vi "Check_Pos_R.vi"(0 "FPGA_Data":sgl[](array[numeric]), 2 "Q_MotorCmd_IN":refnum<queue>, 3 "Q_MotorCmd_Err_IN":errorcluster, 7 "Param_In":T1) -> (6 "LOAD_CELL_PEAK_R":sgl[](array[numeric]), 12 "Target_Pos":i32, 13 "Param_Out":T1, 14 "Flag":T2(ring), 15 "R_NUM":u32, 16 "Q_MotorCmd_OUT":refnum<queue>, 17 "Q_MotorCmd_Err_OUT":errorcluster, 18 "R_Period":u32, 19 "R_GCP":sgl)   [LabVIEW 2019]
uses:
  RT_GLOBAL.vi
panel:
  out "R_Period_EXT":u32
  out "R_GCP_EXT":sgl
  out "R_NUM_EXT":u32
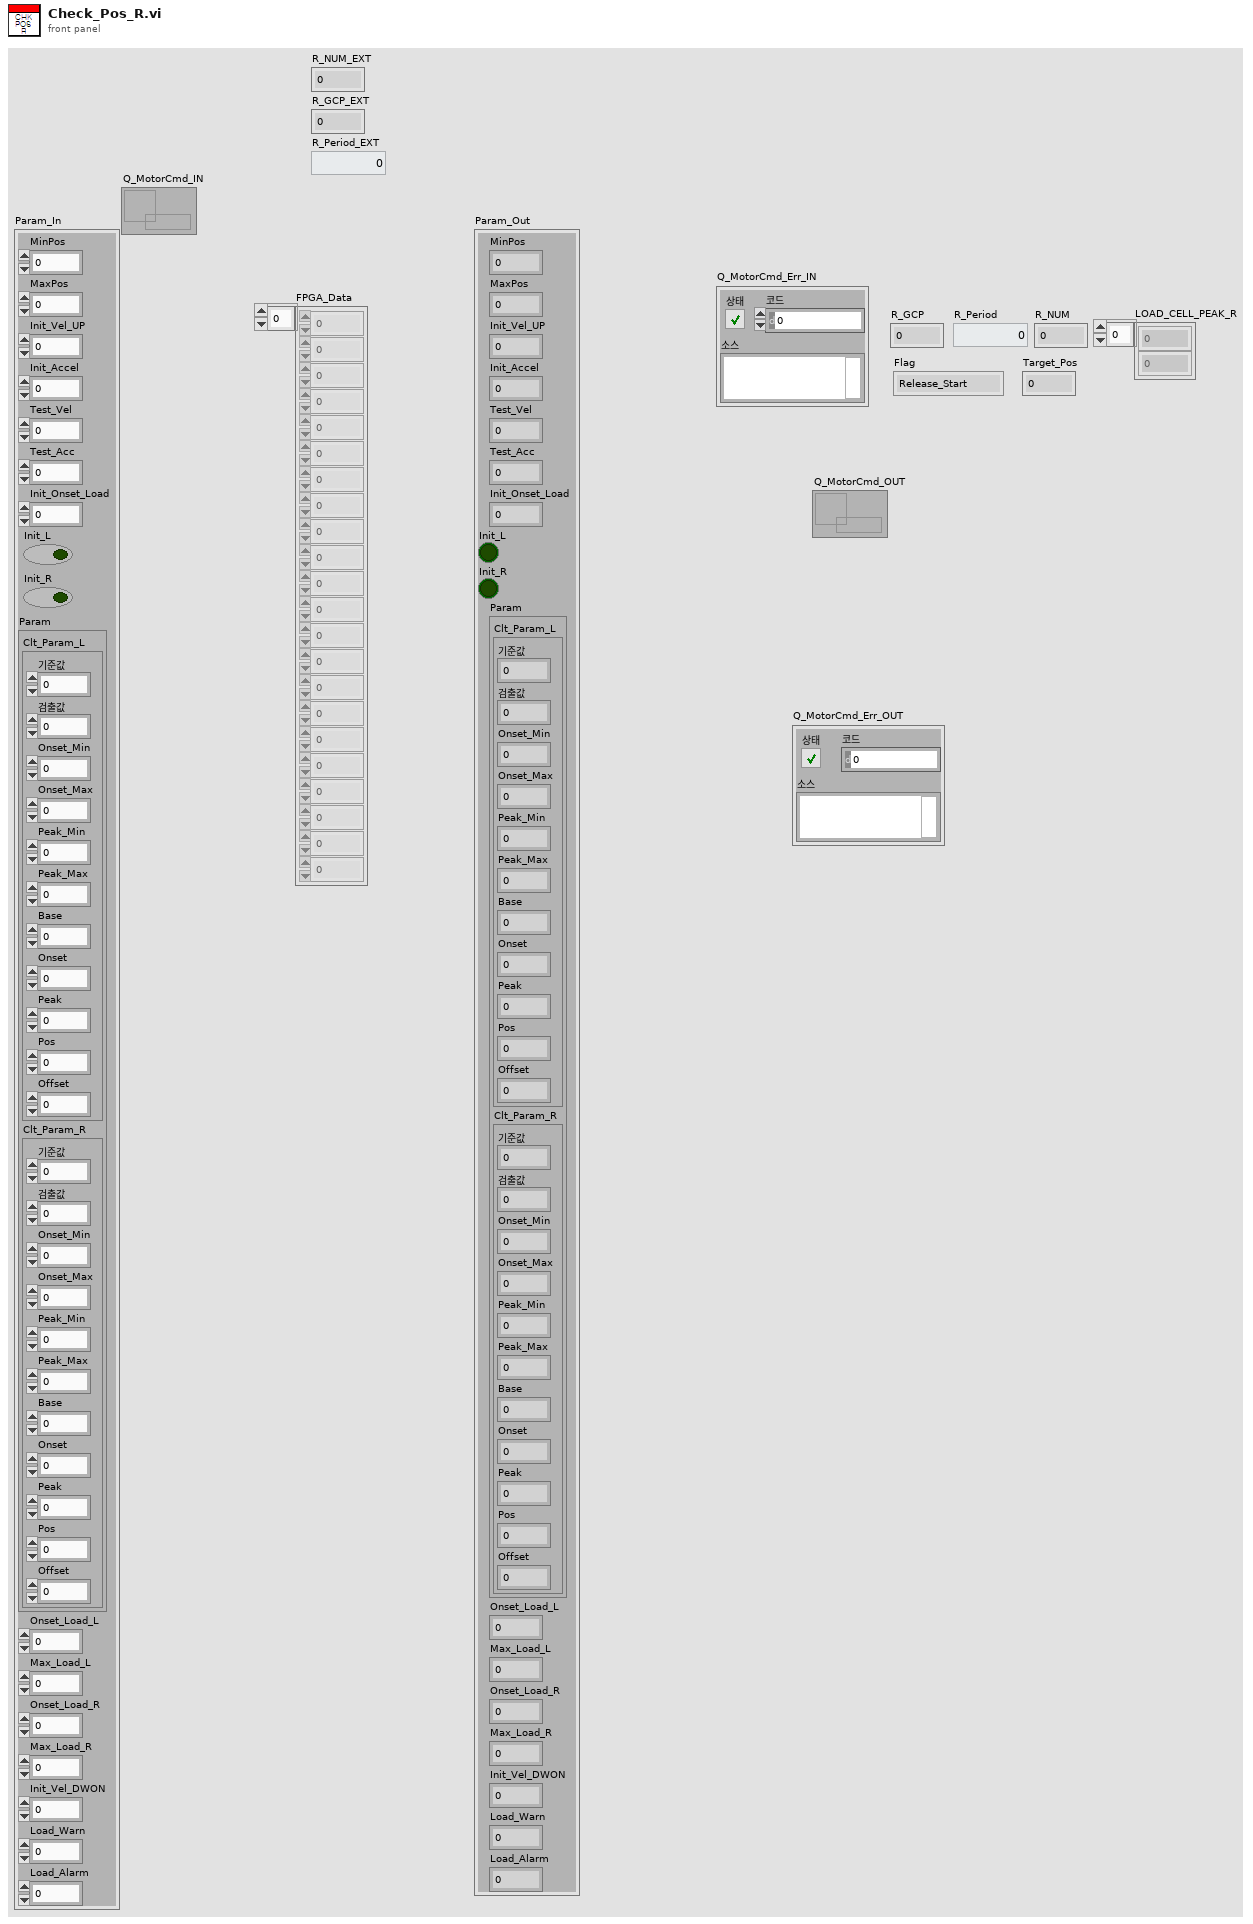
[diagram p1: front panel]
types:
  T1 = cluster{"MinPos":i32, "MaxPos":i32, "Init_Vel_UP":i32, "Init_Accel":u32, "Test_Vel":i32, "Test_Acc":u32, "Init_Onset_Load":sgl, "Init_L":bool, "Init_R":bool, "Param":cluster{"Clt_Param_L":cluster{"기준값":sgl, "검출값":sgl, "Onset_Min":sgl, "Onset_Max":sgl, "Peak_Min":sgl, "Peak_Max":sgl, "Base":i32, "Onset":i32, "Peak":i32, "Pos":i32, "Offset":sgl}, "Clt_Param_R":cluster{"기준값":sgl, "검출값":sgl, "Onset_Min":sgl, "Onset_Max":sgl, "Peak_Min":sgl, "Peak_Max":sgl, "Base":i32, "Onset":i32, "Peak":i32, "Pos":i32, "Offset":sgl}}, "Onset_Load_L":sgl, "Max_Load_L":sgl, "Onset_Load_R":sgl, "Max_Load_R":sgl, "Init_Vel_DWON":i32, "Load_Warn":sgl, "Load_Alarm":sgl}
  T2 = enum16{"Release_Start", "Onset_Start", "Peak_Start", "Calculate"}
  T3 = cluster{"Cmd":string, "Data1":variant, "Data2":variant}
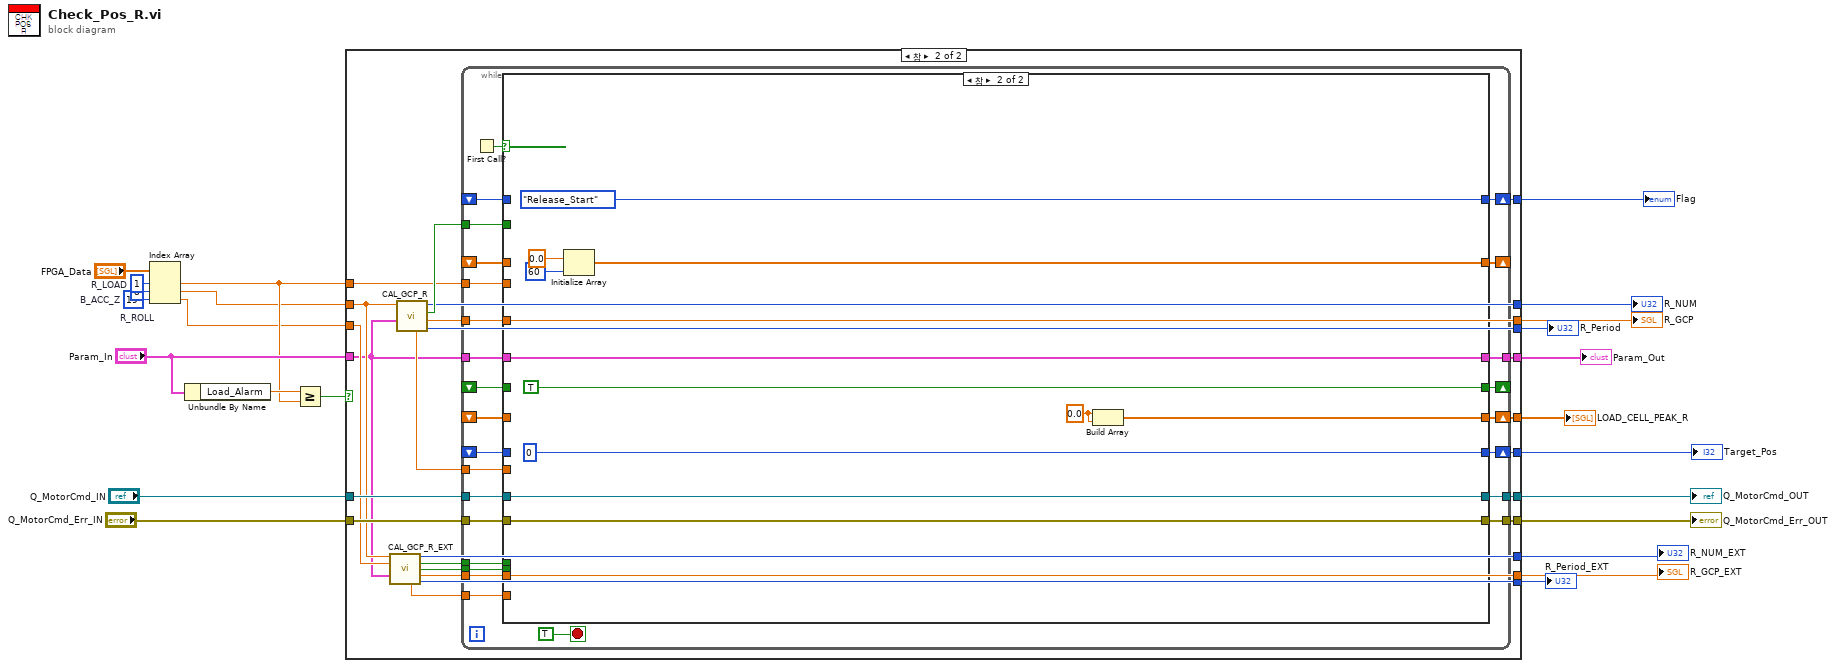
[diagram p0: block diagram]
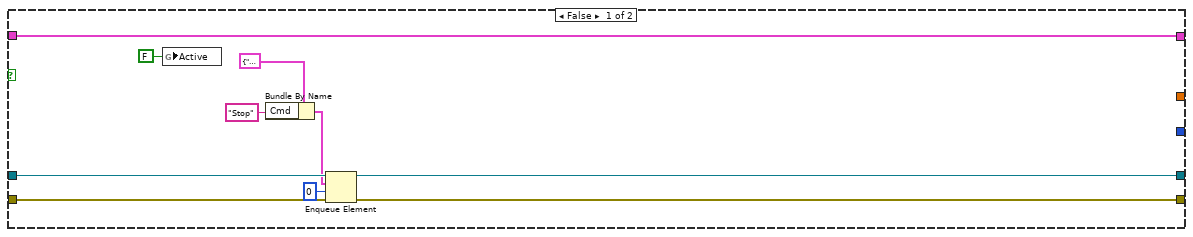
[diagram p2: hidden frame]
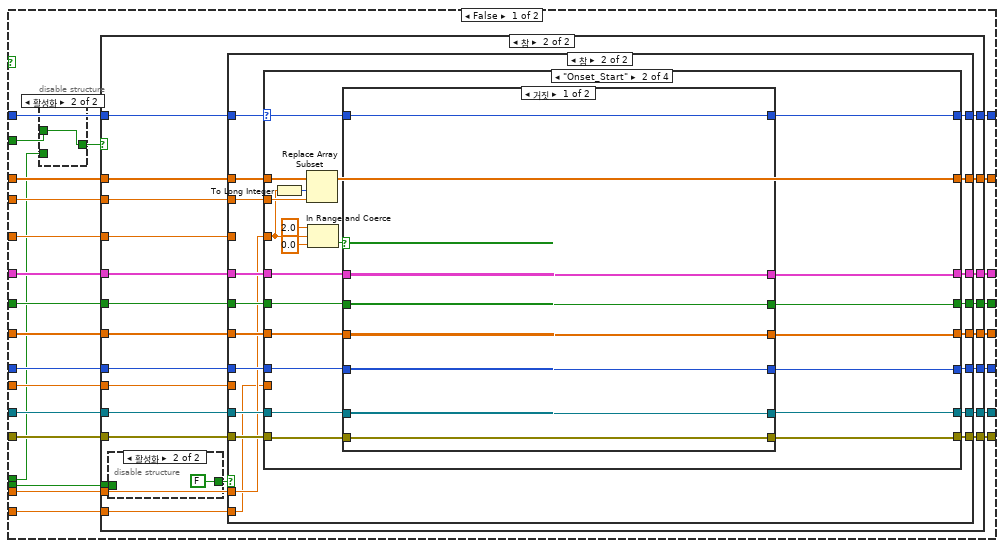
[diagram p3: hidden frame]
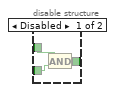
[diagram p4: hidden frame]
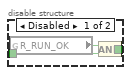
[diagram p6: hidden frame]
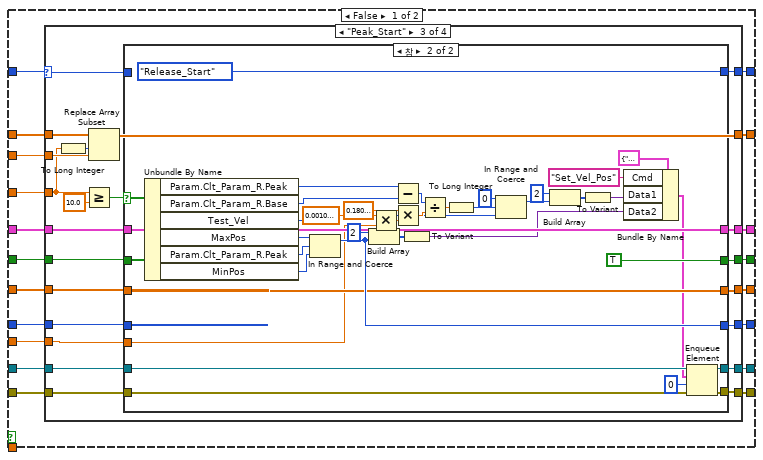
[diagram p7: hidden frame]
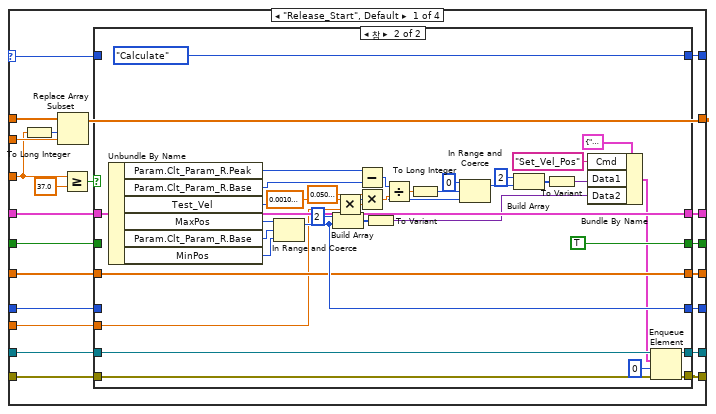
[diagram p8: hidden frame]
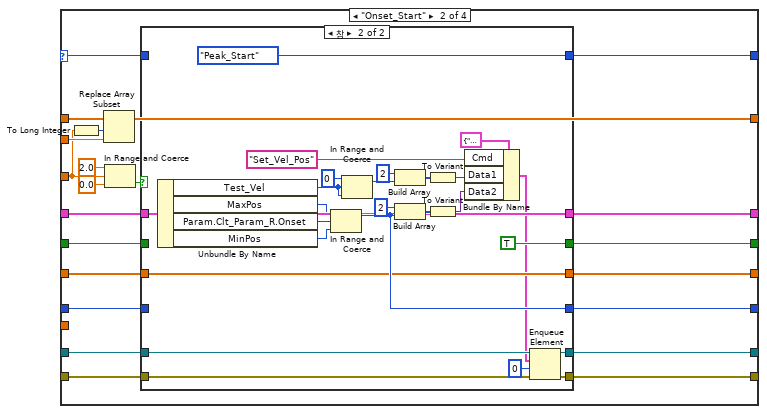
[diagram p10: hidden frame]
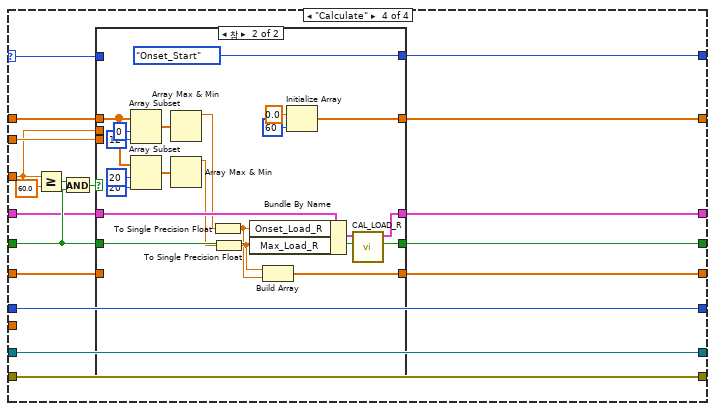
[diagram p13: hidden frame]
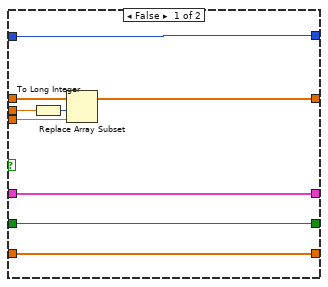
[diagram p14: hidden frame]
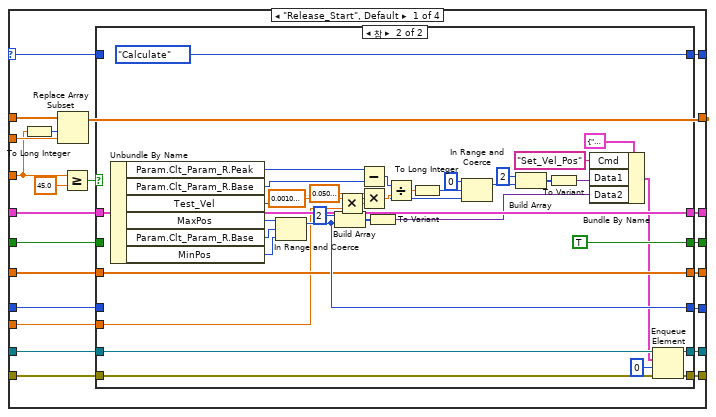
[diagram p15: hidden frame]
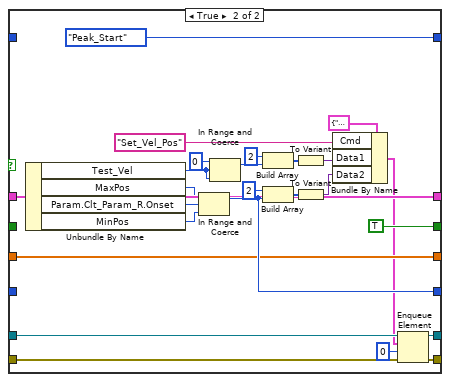
[diagram p17: hidden frame]
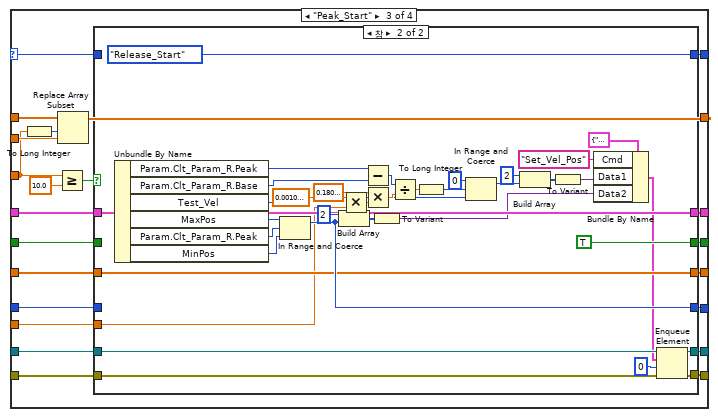
[diagram p18: hidden frame]
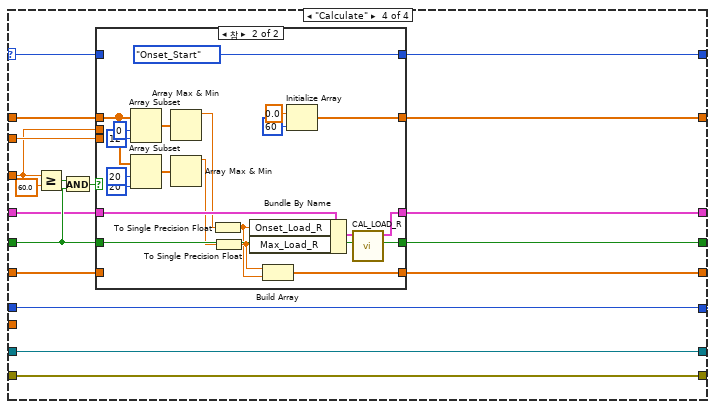
[diagram p20: hidden frame]
diagram:
  w16 = 19  # B_ACC_Z
  w17 = 8  # R_ROLL
  w18 = 1  # R_LOAD
  n1 = Index Array(array="FPGA_Data", index #1=w18, index #2=w17, index #3=w16) -> (element #1=w15:sgl, element #2=w14:sgl, element #3=w13:sgl)
  n2 = Unbundle By Name("Param_In") -> ("Load_Alarm"=w23:sgl)
  n3 = Greater Or Equal?(x=w23, y=w15) -> (x >= y?=w22:bool)
  n4 = case shown="참" w22 {
    tunnel: w14 -> [_ w52]
    tunnel: "Param_In" -> [w27 w50]
    tunnel: "Q_MotorCmd_IN" -> [w31 w56]
    tunnel: "Q_MotorCmd_Err_IN" -> [w30 w55]
    tunnel: w15 -> [_ w54]
    tunnel: w13 -> [_ w51]
    tunnel: [_ w46] -> w12
    tunnel: [_ w45] -> w11
    tunnel: [_ w44] -> w10
    tunnel: [_ w43] -> w9
    tunnel: [w27 w42] -> w8
    tunnel: [_ w41] -> w7
    tunnel: [_ w40] -> w6
    tunnel: [_ w39] -> w5
    tunnel: [_ w38] -> w4
    tunnel: [_ w37] -> w3
    tunnel: [w26 w36] -> w2
    tunnel: [w25 w35] -> w1
    frame False {
      n5 = global write "RT_GLOBAL.vi" "Active"(FALSE ("Active")) -> ()
      n6 = Bundle By Name(cluster=T3 {"Cmd"="", "Data1"=variant, "Data2"=variant}, "Cmd"="Stop") -> (w28:T3)
      n7 = Enqueue Element(queue=w31, element=w28, timeout in ms (-1)=0 ("타임아웃(ms) (-1)"), error in (no error)=w30) -> (queue out=w26:refnum<queue>, error out=w25:errorcluster)  [unwired: 1 out]
    }
    frame True {
      n8 = call "CAL_GCP_R_EXT.vi"("R_ROLL"=w52, "Acc_Z"=w51, "Param_In"=w50) -> ("R_NUM"=w37:u32, "R_Ctrl_Start"=w49:bool, "R_RUN_OK"=w48:bool, "R_GCP_EXT"=w38:sgl, "R_GCP_Total_Time"=w47:sgl, "R_Period"=w39:u32)  [unwired: 7 in]
      n9 = call "CAL_GCP_R.vi"("Param_In"=w50, "R_ROLL"=w52) -> ("R_Period"=w43:u32, "R_GCP"=w44:sgl, "R_Ctrl_Start"=w57:bool, "R_NUM"=w45:u32, "R_GCP_Total_Time"=w53:sgl)  [unwired: 5 in]
      n10 = while {
        tunnel: w57 -> [w81]
        tunnel: w44 -> [w67]
        shift-right: [w82] -> w46
        shift-left: _ -> [w73]
        shift-right: [w80] -> _
        shift-left: _ -> [w72]
        tunnel: w50 -> [w79]
        tunnel: [w78] -> w42
        shift-right: [w76] -> _
        shift-left: _ -> [w77]
        shift-right: [w75] -> w40
        shift-left: _ -> [w70]
        tunnel: w56 -> [w69]
        tunnel: w55 -> [w68]
        tunnel: w54 -> [w71]
        shift-right: [w66] -> w41
        shift-left: _ -> [w65]
        tunnel: w53 -> [w64]
        tunnel: w49 -> [w63]
        tunnel: w48 -> [w62]
        tunnel: w38 -> [w61]
        tunnel: w47 -> [w60]
        tunnel: [w59] -> w36
        tunnel: [w58] -> w35
        stop <- TRUE stop-if-true
        n11 = First Call?() -> (First Call?: T/F=w83:bool)
        n12 = case shown="참" w83 {
          tunnel: [w108 T2."Release_Start"] -> w82
          tunnel: w81 -> [w91 _]
          tunnel: [w105 w651] -> w80
          tunnel: [w102 w650] -> w78
          tunnel: w79 -> [w103 w650]
          tunnel: w77 -> [w100 _]
          tunnel: [w101 TRUE] -> w76
          tunnel: [w98 0] -> w75
          tunnel: w73 -> [w107 _]
          tunnel: w72 -> [w106 _]
          tunnel: w71 -> [w104 _]
          tunnel: w70 -> [w99 _]
          tunnel: w69 -> [w97 w645]
          tunnel: w68 -> [w96 w644]
          tunnel: w67 -> [w95 _]
          tunnel: [w94 w647] -> w66
          tunnel: w65 -> [w93 _]
          tunnel: w64 -> [w92 _]
          tunnel: w63 -> [w90 _]
          tunnel: w62 -> [w88 _]
          tunnel: w61 -> [w87 _]
          tunnel: w60 -> [w86 _]
          tunnel: [w85 w645] -> w59
          tunnel: [w84 w644] -> w58
          frame False {
            n13 = disable-structure shown="활성화" {
              disable-tunnel: w91 -> [w111 w112]
              disable-tunnel: w90 -> [w110 _]
              disable-tunnel: [w109 w112] -> w89
              frame Disabled {
                n14 = And(x=w111, y=w110) -> (x .and. y?=w109:bool)
              }
              frame Enabled {
              }
            }
            n15 = case shown="참" w89 {
              tunnel: [w120 w142] -> w108
              tunnel: w107 -> [w120 w143]
              tunnel: [w119 w140] -> w105
              tunnel: w106 -> [w119 w141]
              tunnel: w104 -> [_ w138]
              tunnel: [w118 w136] -> w102
              tunnel: w103 -> [w118 w137]
              tunnel: [w117 w135] -> w101
              tunnel: w100 -> [w117 w134]
              tunnel: [w116 w133] -> w98
              tunnel: w99 -> [w116 w132]
              tunnel: w97 -> [w114 w131]
              tunnel: w96 -> [w113 w130]
              tunnel: w95 -> [_ w139]
              tunnel: [w115 w129] -> w94
              tunnel: w93 -> [w115 w128]
              tunnel: w92 -> [_ w127]
              tunnel: w88 -> [_ w126]
              tunnel: w87 -> [_ w124]
              tunnel: w86 -> [_ w123]
              tunnel: [w114 w122] -> w85
              tunnel: [w113 w121] -> w84
              frame False {
              }
              frame True {
                n16 = disable-structure shown="활성화" {
                  disable-tunnel: w126 -> [w146 _]
                  disable-tunnel: [w144 FALSE] -> w125
                  frame Disabled {
                    n17 = global read "RT_GLOBAL.vi" "R_RUN_OK"() -> (w145:bool)
                    n18 = And(x=w145, y=w146) -> (x .and. y?=w144:bool)
                  }
                  frame Enabled {
                  }
                }
                n19 = case shown="참" w125 {
                  tunnel: w143 -> [w166 w414]
                  tunnel: [w165 w413] -> w142
                  tunnel: w141 -> [w164 w412]
                  tunnel: [w163 w411] -> w140
                  tunnel: w139 -> [w162 _]
                  tunnel: w138 -> [w161 w410]
                  tunnel: w137 -> [w160 w409]
                  tunnel: [w159 w408] -> w136
                  tunnel: [w158 w407] -> w135
                  tunnel: w134 -> [w157 w406]
                  tunnel: [w156 w405] -> w133
                  tunnel: w132 -> [w155 w404]
                  tunnel: w131 -> [w154 w403]
                  tunnel: w130 -> [w153 w402]
                  tunnel: [w152 w401] -> w129
                  tunnel: w128 -> [w151 w400]
                  tunnel: w127 -> [w150 _]
                  tunnel: w124 -> [_ w399]
                  tunnel: w123 -> [_ w398]
                  tunnel: [w149 w397] -> w122
                  tunnel: [w148 w396] -> w121
                  frame False {
                    n20 = case shown="\"Peak_Start\"" w166 {
                      selector: w166 -> [w186 w252 w300 w366]
                      tunnel: [w176 w251 w285 w365] -> w165
                      tunnel: w164 -> [w185 w247 w305 w364]
                      tunnel: [w177 w246 w304 w363] -> w163
                      tunnel: w162 -> [w178 w244 w301 w360]
                      tunnel: w161 -> [w184 w245 w302 w362]
                      tunnel: w160 -> [w183 w243 w298 w354]
                      tunnel: [w175 w242 w291 w353] -> w159
                      tunnel: [w174 w241 w286 w358] -> w158
                      tunnel: w157 -> [w182 w240 w297 w357]
                      tunnel: [w173 w239 w288 w355] -> w156
                      tunnel: w155 -> [w181 w238 w295 w355]
                      tunnel: w154 -> [w180 w237 w293 w350]
                      tunnel: w153 -> [w179 w236 w292 w349]
                      tunnel: [w171 w234 w287 w352] -> w152
                      tunnel: w151 -> [w172 w235 w296 w351]
                      tunnel: w150 -> [w170 _ w294 _]
                      tunnel: [w168 w232 w290 w350] -> w149
                      tunnel: [w167 w231 w289 w349] -> w148
                      frame "Release_Start", Default {
                        n21 = To Long Integer(number=w178) -> (32bit integer=w187:i32)
                        n22 = Replace Array Subset(array=w185, new element=w184, index=w187) -> (w177:sgl[])
                        n23 = Greater Or Equal?(x=w178, y=sgl 37.0) -> (x >= y?=w169:bool)
                        n24 = case shown="참" w169 {
                          tunnel: w186 -> [w195 _]
                          tunnel: [w195 T2."Calculate"] -> w176
                          tunnel: [w194 w212] -> w175
                          tunnel: w183 -> [w194 w212]
                          tunnel: [w193 TRUE] -> w174
                          tunnel: w182 -> [w193 _]
                          tunnel: [w192 w227] -> w173
                          tunnel: w181 -> [w192 _]
                          tunnel: w180 -> [w190 w210]
                          tunnel: w179 -> [w189 w211]
                          tunnel: w172 -> [w191 w225]
                          tunnel: [w191 w225] -> w171
                          tunnel: w170 -> [_ w205]
                          tunnel: [w190 w198] -> w168
                          tunnel: [w189 w197] -> w167
                          frame False {
                          }
                          frame True {
                            n25 = Unbundle By Name(w212) -> ("Param.Clt_Param_R.Peak"=w220:i32, "Param.Clt_Param_R.Base"=w221:i32, "Test_Vel"=w196:i32, "MaxPos"=w201:i32, "Param.Clt_Param_R.Base"=w200:i32, "MinPos"=w199:i32)
                            n26 = In Range and Coerce(upper limit=w201, x=w200, lower limit=w199) -> (coerced(x)=w227:i32)  [unwired: 1 out]
                            n27 = Build Array(2 ("원소"), w227) -> (w229:i32[])
                            n28 = Multiply(x=sgl 0.001 ("y"), y=w205) -> (x*y=w203:sgl)
                            n29 = Subtract(x=w220, y=w221) -> (x-y=w222:i32)
                            n30 = Multiply(x=sgl 0.05 ("y"), y=w203) -> (x*y=w217:sgl)
                            n31 = To Variant(anything=w229) -> (Variant=w206:variant)
                            n32 = Divide(x=w222, y=w217) -> (x/y=w223:sgl)
                            n33 = To Long Integer(number=w223) -> (32bit integer=w209:i32)
                            n34 = In Range and Coerce(upper limit=0, x=w209, lower limit=w196) -> (coerced(x)=w224:i32)  [unwired: 1 out]
                            n35 = Build Array(2 ("원소"), w224) -> (w219:i32[])
                            n36 = To Variant(anything=w219) -> (Variant=w218:variant)
                            n37 = Bundle By Name(cluster=T3 {"Cmd"="", "Data1"=variant, "Data2"=variant}, "Cmd"="Set_Vel_Pos", "Data1"=w218, "Data2"=w206) -> (w207:T3)
                            n38 = Enqueue Element(queue=w210, element=w207, timeout in ms (-1)=0 ("타임아웃(ms) (-1)"), error in (no error)=w211) -> (queue out=w198:refnum<queue>, error out=w197:errorcluster)  [unwired: 1 out]
                          }
                        }
                      }
                      frame "Onset_Start" {
                        n39 = To Long Integer(number=w244) -> (32bit integer=w248:i32)
                        n40 = Replace Array Subset(array=w247, new element=w245, index=w248) -> (w246:sgl[])
                        n41 = In Range and Coerce(upper limit=sgl 2.0 ("상위 리미트"), x=w244, lower limit=sgl 0.0 ("하위 리미트")) -> (In Range?=w233:bool)  [unwired: 1 out]
                        n42 = case shown="참" w233 {
                          tunnel: w252 -> [w259 _]
                          tunnel: [w259 T2."Peak_Start"] -> w251
                          tunnel: [w258 w269] -> w242
                          tunnel: w243 -> [w258 w269]
                          tunnel: [w257 TRUE] -> w241
                          tunnel: w240 -> [w257 _]
                          tunnel: [w256 w281] -> w239
                          tunnel: w238 -> [w256 _]
                          tunnel: w237 -> [w254 w271]
                          tunnel: w236 -> [w253 w270]
                          tunnel: [w255 w279] -> w234
                          tunnel: w235 -> [w255 w279]
                          tunnel: [w254 w261] -> w232
                          tunnel: [w253 w260] -> w231
                          frame False {
                          }
                          frame True {
                            n43 = Unbundle By Name(w269) -> ("Test_Vel"=w268:i32, "MaxPos"=w264:i32, "Param.Clt_Param_R.Onset"=w263:i32, "MinPos"=w262:i32)
                            n44 = In Range and Coerce(upper limit=w264, x=w263, lower limit=w262) -> (coerced(x)=w281:i32)  [unwired: 1 out]
                            n45 = In Range and Coerce(upper limit=0, x=w268, lower limit=w268) -> (coerced(x)=w278:i32)  [unwired: 1 out]
                            n46 = Build Array(2 ("원소"), w278) -> (w277:i32[])
                            n47 = Build Array(2 ("원소"), w281) -> (w283:i32[])
                            n48 = To Variant(anything=w277) -> (Variant=w276:variant)
                            n49 = To Variant(anything=w283) -> (Variant=w265:variant)
                            n50 = Bundle By Name(cluster=T3 {"Cmd"="", "Data1"=variant, "Data2"=variant}, "Cmd"="Set_Vel_Pos", "Data1"=w276, "Data2"=w265) -> (w266:T3)
                            n51 = Enqueue Element(queue=w271, element=w266, timeout in ms (-1)=0 ("타임아웃(ms) (-1)"), error in (no error)=w270) -> (queue out=w261:refnum<queue>, error out=w260:errorcluster)  [unwired: 1 out]
                          }
                        }
                      }
                      frame "Peak_Start" {
                        n52 = To Long Integer(number=w301) -> (32bit integer=w303:i32)
                        n53 = Greater Or Equal?(x=w301, y=sgl 10.0) -> (x >= y?=w299:bool)
                        n54 = Replace Array Subset(array=w305, new element=w302, index=w303) -> (w304:sgl[])
                        n55 = case shown="참" w299 {
                          tunnel: w300 -> [w313 _]
                          tunnel: [w313 T2."Release_Start"] -> w285
                          tunnel: [w312 w330] -> w291
                          tunnel: w298 -> [w312 w330]
                          tunnel: [w311 TRUE] -> w286
                          tunnel: w297 -> [w311 _]
                          tunnel: [w310 w345] -> w288
                          tunnel: w295 -> [w310 _]
                          tunnel: w293 -> [w308 w328]
                          tunnel: w292 -> [w307 w329]
                          tunnel: w296 -> [w309 w343]
                          tunnel: [w309 w343] -> w287
                          tunnel: w294 -> [_ w323]
                          tunnel: [w308 w316] -> w290
                          tunnel: [w307 w315] -> w289
                          frame False {
                          }
                          frame True {
                            n56 = Unbundle By Name(w330) -> ("Param.Clt_Param_R.Peak"=w338:i32, "Param.Clt_Param_R.Base"=w339:i32, "Test_Vel"=w314:i32, "MaxPos"=w319:i32, "Param.Clt_Param_R.Peak"=w318:i32, "MinPos"=w317:i32)
                            n57 = In Range and Coerce(upper limit=w319, x=w318, lower limit=w317) -> (coerced(x)=w345:i32)  [unwired: 1 out]
                            n58 = Build Array(2 ("원소"), w345) -> (w347:i32[])
                            n59 = Multiply(x=sgl 0.001 ("y"), y=w323) -> (x*y=w321:sgl)
                            n60 = Subtract(x=w338, y=w339) -> (x-y=w340:i32)
                            n61 = Multiply(x=sgl 0.18 ("y"), y=w321) -> (x*y=w335:sgl)
                            n62 = To Variant(anything=w347) -> (Variant=w324:variant)
                            n63 = Divide(x=w340, y=w335) -> (x/y=w341:sgl)
                            n64 = To Long Integer(number=w341) -> (32bit integer=w327:i32)
                            n65 = In Range and Coerce(upper limit=0, x=w327, lower limit=w314) -> (coerced(x)=w342:i32)  [unwired: 1 out]
                            n66 = Build Array(2 ("원소"), w342) -> (w337:i32[])
                            n67 = To Variant(anything=w337) -> (Variant=w336:variant)
                            n68 = Bundle By Name(cluster=T3 {"Cmd"="", "Data1"=variant, "Data2"=variant}, "Cmd"="Set_Vel_Pos", "Data1"=w336, "Data2"=w324) -> (w325:T3)
                            n69 = Enqueue Element(queue=w328, element=w325, timeout in ms (-1)=0 ("타임아웃(ms) (-1)"), error in (no error)=w329) -> (queue out=w316:refnum<queue>, error out=w315:errorcluster)  [unwired: 1 out]
                          }
                        }
                      }
                      frame "Calculate" {
                        n70 = Greater Or Equal?(x=w360, y=sgl 60.0) -> (x >= y?=w359:bool)
                        n71 = And(x=w359, y=w357) -> (x .and. y?=w356:bool)
                        n72 = case shown="참" w356 {
                          tunnel: [w375 T2."Onset_Start"] -> w365
                          tunnel: w366 -> [w375 _]
                          tunnel: w364 -> [w373 w387]
                          tunnel: [w372 w392] -> w363
                          tunnel: w360 -> [w371 _]
                          tunnel: w362 -> [w370 _]
                          tunnel: [w369 w391] -> w358
                          tunnel: w357 -> [w369 w391]
                          tunnel: w354 -> [w368 w390]
                          tunnel: [w368 w388] -> w353
                          tunnel: [w367 w376] -> w352
                          tunnel: w351 -> [w367 _]
                          frame False {
                            n73 = To Long Integer(number=w371) -> (32bit integer=w374:i32)
                            n74 = Replace Array Subset(array=w373, new element=w370, index=w374) -> (w372:sgl[])
                          }
                          frame True {
                            n75 = Array Subset(array=w387, index=0 ("인덱스"), length=12 ("길이")) -> (w386:sgl[])
                            n76 = Array Subset(array=w387, index=20 ("인덱스"), length=20 ("길이")) -> (w385:sgl[])
                            n77 = Array Max & Min(array=w386) -> (max value=w380:sgl)  [unwired: 3 out]
                            n78 = Array Max & Min(array=w385) -> (max value=w379:sgl)  [unwired: 3 out]
                            n79 = To Single Precision Float(number=w380) -> (single precision float=w377:sgl)
                            n80 = To Single Precision Float(number=w379) -> (single precision float=w378:sgl)
                            n81 = Bundle By Name(cluster=w390, "Onset_Load_R"=w377, "Max_Load_R"=w378) -> (w389:T1)
                            n82 = Build Array(w378, w377) -> (w376:sgl[])
                            n83 = Initialize Array(sgl 0.0 ("원소"), 60 ("차원 크기")) -> (w392:sgl[])
                            n84 = call "CAL_LOAD_R.vi"("Param_In"=w389) -> ("Param_Out"=w388:T1)  [unwired: 10 in]
                          }
                        }
                      }
                    }
                  }
                  frame True {
                    n85 = case shown="\"Onset_Start\"" w414 {
                      selector: w414 -> [w430 w493 w548 w614]
                      tunnel: [w421 w492 w545 w613] -> w413
                      tunnel: w412 -> [w434 w497 w553 w612]
                      tunnel: [w431 w496 w552 w611] -> w411
                      tunnel: w399 -> [w432 w494 w549 w608]
                      tunnel: w410 -> [w433 w495 w550 w610]
                      tunnel: w409 -> [w428 w490 w546 w602]
                      tunnel: [w418 w479 w538 w601] -> w408
                      tunnel: [w417 w480 w536 w606] -> w407
                      tunnel: w406 -> [w427 w489 w544 w605]
                      tunnel: [w415 w482 w535 w603] -> w405
                      tunnel: w404 -> [w425 w487 w542 w603]
                      tunnel: w403 -> [w423 w486 w540 w598]
                      tunnel: w402 -> [w422 w485 w539 w597]
                      tunnel: [w416 w481 w537 w600] -> w401
                      tunnel: w400 -> [w426 w488 w543 w599]
                      tunnel: w398 -> [w424 _ w541 _]
                      tunnel: [w420 w484 w534 w598] -> w397
                      tunnel: [w419 w483 w533 w597] -> w396
                      frame "Release_Start", Default {
                        n86 = To Long Integer(number=w432) -> (32bit integer=w435:i32)
                        n87 = Replace Array Subset(array=w434, new element=w433, index=w435) -> (w431:sgl[])
                        n88 = Greater Or Equal?(x=w432, y=sgl 45.0) -> (x >= y?=w429:bool)
                        n89 = case shown="참" w429 {
                          tunnel: w430 -> [w443 _]
                          tunnel: [w443 T2."Calculate"] -> w421
                          tunnel: [w442 w460] -> w418
                          tunnel: w428 -> [w442 w460]
                          tunnel: [w441 TRUE] -> w417
                          tunnel: w427 -> [w441 _]
                          tunnel: [w440 w475] -> w415
                          tunnel: w425 -> [w440 _]
                          tunnel: w423 -> [w438 w458]
                          tunnel: w422 -> [w437 w459]
                          tunnel: w426 -> [w439 w473]
                          tunnel: [w439 w473] -> w416
                          tunnel: w424 -> [_ w453]
                          tunnel: [w438 w446] -> w420
                          tunnel: [w437 w445] -> w419
                          frame False {
                          }
                          frame True {
                            n90 = Unbundle By Name(w460) -> ("Param.Clt_Param_R.Peak"=w468:i32, "Param.Clt_Param_R.Base"=w469:i32, "Test_Vel"=w444:i32, "MaxPos"=w449:i32, "Param.Clt_Param_R.Base"=w448:i32, "MinPos"=w447:i32)
                            n91 = In Range and Coerce(upper limit=w449, x=w448, lower limit=w447) -> (coerced(x)=w475:i32)  [unwired: 1 out]
                            n92 = Build Array(2 ("원소"), w475) -> (w477:i32[])
                            n93 = Multiply(x=sgl 0.001 ("y"), y=w453) -> (x*y=w451:sgl)
                            n94 = Subtract(x=w468, y=w469) -> (x-y=w470:i32)
                            n95 = Multiply(x=sgl 0.05 ("y"), y=w451) -> (x*y=w465:sgl)
                            n96 = To Variant(anything=w477) -> (Variant=w454:variant)
                            n97 = Divide(x=w470, y=w465) -> (x/y=w471:sgl)
                            n98 = To Long Integer(number=w471) -> (32bit integer=w457:i32)
                            n99 = In Range and Coerce(upper limit=0, x=w457, lower limit=w444) -> (coerced(x)=w472:i32)  [unwired: 1 out]
                            n100 = Build Array(2 ("원소"), w472) -> (w467:i32[])
                            n101 = To Variant(anything=w467) -> (Variant=w466:variant)
                            n102 = Bundle By Name(cluster=T3 {"Cmd"="", "Data1"=variant, "Data2"=variant}, "Cmd"="Set_Vel_Pos", "Data1"=w466, "Data2"=w454) -> (w455:T3)
                            n103 = Enqueue Element(queue=w458, element=w455, timeout in ms (-1)=0 ("타임아웃(ms) (-1)"), error in (no error)=w459) -> (queue out=w446:refnum<queue>, error out=w445:errorcluster)  [unwired: 1 out]
                          }
                        }
                      }
                      frame "Onset_Start" {
                        n104 = To Long Integer(number=w494) -> (32bit integer=w498:i32)
                        n105 = Replace Array Subset(array=w497, new element=w495, index=w498) -> (w496:sgl[])
                        n106 = In Range and Coerce(upper limit=sgl 2.0 ("상위 리미트"), x=w494, lower limit=sgl 0.0 ("하위 리미트")) -> (In Range?=w491:bool)  [unwired: 1 out]
                        n107 = case shown="거짓" w491 {
                          tunnel: w493 -> [w507 _]
                          tunnel: [w507 T2."Peak_Start"] -> w492
                          tunnel: [w506 w517] -> w479
                          tunnel: w490 -> [w506 w517]
                          tunnel: [w505 TRUE] -> w480
                          tunnel: w489 -> [w505 _]
                          tunnel: [w504 w529] -> w482
                          tunnel: w487 -> [w504 _]
                          tunnel: w486 -> [w502 w519]
                          tunnel: w485 -> [w501 w518]
                          tunnel: [w503 w527] -> w481
                          tunnel: w488 -> [w503 w527]
                          tunnel: [w502 w509] -> w484
                          tunnel: [w501 w508] -> w483
                          frame False {
                          }
                          frame True {
                            n108 = Unbundle By Name(w517) -> ("Test_Vel"=w516:i32, "MaxPos"=w512:i32, "Param.Clt_Param_R.Onset"=w511:i32, "MinPos"=w510:i32)
                            n109 = In Range and Coerce(upper limit=w512, x=w511, lower limit=w510) -> (coerced(x)=w529:i32)  [unwired: 1 out]
                            n110 = In Range and Coerce(upper limit=0, x=w516, lower limit=w516) -> (coerced(x)=w526:i32)  [unwired: 1 out]
                            n111 = Build Array(2 ("원소"), w526) -> (w525:i32[])
                            n112 = Build Array(2 ("원소"), w529) -> (w531:i32[])
                            n113 = To Variant(anything=w525) -> (Variant=w524:variant)
                            n114 = To Variant(anything=w531) -> (Variant=w513:variant)
                            n115 = Bundle By Name(cluster=T3 {"Cmd"="", "Data1"=variant, "Data2"=variant}, "Cmd"="Set_Vel_Pos", "Data1"=w524, "Data2"=w513) -> (w514:T3)
                            n116 = Enqueue Element(queue=w519, element=w514, timeout in ms (-1)=0 ("타임아웃(ms) (-1)"), error in (no error)=w518) -> (queue out=w509:refnum<queue>, error out=w508:errorcluster)  [unwired: 1 out]
                          }
                        }
                      }
                      frame "Peak_Start" {
                        n117 = To Long Integer(number=w549) -> (32bit integer=w551:i32)
                        n118 = Greater Or Equal?(x=w549, y=sgl 10.0) -> (x >= y?=w547:bool)
                        n119 = Replace Array Subset(array=w553, new element=w550, index=w551) -> (w552:sgl[])
                        n120 = case shown="참" w547 {
                          tunnel: w548 -> [w561 _]
                          tunnel: [w561 T2."Release_Start"] -> w545
                          tunnel: [w560 w578] -> w538
                          tunnel: w546 -> [w560 w578]
                          tunnel: [w559 TRUE] -> w536
                          tunnel: w544 -> [w559 _]
                          tunnel: [w558 w593] -> w535
                          tunnel: w542 -> [w558 _]
                          tunnel: w540 -> [w556 w576]
                          tunnel: w539 -> [w555 w577]
                          tunnel: w543 -> [w557 w591]
                          tunnel: [w557 w591] -> w537
                          tunnel: w541 -> [_ w571]
                          tunnel: [w556 w564] -> w534
                          tunnel: [w555 w563] -> w533
                          frame False {
                          }
                          frame True {
                            n121 = Unbundle By Name(w578) -> ("Param.Clt_Param_R.Peak"=w586:i32, "Param.Clt_Param_R.Base"=w587:i32, "Test_Vel"=w562:i32, "MaxPos"=w567:i32, "Param.Clt_Param_R.Peak"=w566:i32, "MinPos"=w565:i32)
                            n122 = In Range and Coerce(upper limit=w567, x=w566, lower limit=w565) -> (coerced(x)=w593:i32)  [unwired: 1 out]
                            n123 = Build Array(2 ("원소"), w593) -> (w595:i32[])
                            n124 = Multiply(x=sgl 0.001 ("y"), y=w571) -> (x*y=w569:sgl)
                            n125 = Subtract(x=w586, y=w587) -> (x-y=w588:i32)
                            n126 = Multiply(x=sgl 0.18 ("y"), y=w569) -> (x*y=w583:sgl)
                            n127 = To Variant(anything=w595) -> (Variant=w572:variant)
                            n128 = Divide(x=w588, y=w583) -> (x/y=w589:sgl)
                            n129 = To Long Integer(number=w589) -> (32bit integer=w575:i32)
                            n130 = In Range and Coerce(upper limit=0, x=w575, lower limit=w562) -> (coerced(x)=w590:i32)  [unwired: 1 out]
                            n131 = Build Array(2 ("원소"), w590) -> (w585:i32[])
                            n132 = To Variant(anything=w585) -> (Variant=w584:variant)
                            n133 = Bundle By Name(cluster=T3 {"Cmd"="", "Data1"=variant, "Data2"=variant}, "Cmd"="Set_Vel_Pos", "Data1"=w584, "Data2"=w572) -> (w573:T3)
                            n134 = Enqueue Element(queue=w576, element=w573, timeout in ms (-1)=0 ("타임아웃(ms) (-1)"), error in (no error)=w577) -> (queue out=w564:refnum<queue>, error out=w563:errorcluster)  [unwired: 1 out]
                          }
                        }
                      }
                      frame "Calculate" {
                        n135 = Greater Or Equal?(x=w608, y=sgl 60.0) -> (x >= y?=w607:bool)
                        n136 = And(x=w607, y=w605) -> (x .and. y?=w604:bool)
                        n137 = case shown="참" w604 {
                          tunnel: [w623 T2."Onset_Start"] -> w613
                          tunnel: w614 -> [w623 _]
                          tunnel: w612 -> [w621 w635]
                          tunnel: [w620 w640] -> w611
                          tunnel: w608 -> [w619 _]
                          tunnel: w610 -> [w618 _]
                          tunnel: [w617 w639] -> w606
                          tunnel: w605 -> [w617 w639]
                          tunnel: w602 -> [w616 w638]
                          tunnel: [w616 w636] -> w601
                          tunnel: [w615 w624] -> w600
                          tunnel: w599 -> [w615 _]
                          frame False {
                            n138 = To Long Integer(number=w619) -> (32bit integer=w622:i32)
                            n139 = Replace Array Subset(array=w621, new element=w618, index=w622) -> (w620:sgl[])
                          }
                          frame True {
                            n140 = Array Subset(array=w635, index=0 ("인덱스"), length=12 ("길이")) -> (w634:sgl[])
                            n141 = Array Subset(array=w635, index=20 ("인덱스"), length=20 ("길이")) -> (w633:sgl[])
                            n142 = Array Max & Min(array=w634) -> (max value=w628:sgl)  [unwired: 3 out]
                            n143 = Array Max & Min(array=w633) -> (max value=w627:sgl)  [unwired: 3 out]
                            n144 = To Single Precision Float(number=w628) -> (single precision float=w625:sgl)
                            n145 = To Single Precision Float(number=w627) -> (single precision float=w626:sgl)
                            n146 = Bundle By Name(cluster=w638, "Onset_Load_R"=w625, "Max_Load_R"=w626) -> (w637:T1)
                            n147 = Build Array(w626, w625) -> (w624:sgl[])
                            n148 = Initialize Array(sgl 0.0 ("원소"), 60 ("차원 크기")) -> (w640:sgl[])
                            n149 = call "CAL_LOAD_R.vi"("Param_In"=w637) -> ("Param_Out"=w636:T1)  [unwired: 10 in]
                          }
                        }
                      }
                    }
                  }
                }
              }
            }
          }
          frame True {
            w646 = sgl 0.0 ("원소")
            n150 = Initialize Array(sgl 0.0 ("원소"), 60 ("차원 크기")) -> (w651:sgl[])
            n151 = Build Array(w646, w646) -> (w647:sgl[])
          }
        }
      }
    }
  }
  "Flag" <- w12
  "R_NUM" <- w11
  "R_GCP" <- w10
  "R_Period" <- w9
  "Param_Out" <- w8
  "LOAD_CELL_PEAK_R" <- w7
  "Target_Pos" <- w6
  "R_NUM_EXT" <- w3
  "R_GCP_EXT" <- w4
  "R_Period_EXT" <- w5
  "Q_MotorCmd_Err_OUT" <- w1
  "Q_MotorCmd_OUT" <- w2
